vi "test-sync response for csm loop.vi"(8 "error in (no error)":errorcluster, 11 "TestCase in":refnum<class "testcase-csm loop support.lvclass">) -> (0 "error out":errorcluster, 3 "TestCase out":refnum<class "testcase-csm loop support.lvclass">)   [LabVIEW 2017, in "testcase-csm loop support.lvclass"]
uses:
  testcase-csm loop support.lvclass
  56d4bdba-c2f1-4b55-add1-7a078de9da03.vi
  ea54eaf7-6c78-4206-8259-080cdfbb85de.vi
  src/user.lib/_NEVSTOP/Communicable State Machine(CSM)/AdvanceAPI/CSM - Revert Arguments-Safe String.vi
  src/user.lib/_NEVSTOP/Communicable State Machine(CSM)/AdvanceAPI/CSM - Make String Arguments Safe.vi
  src/user.lib/_NEVSTOP/Communicable State Machine(CSM)/AdvanceAPI/CSM - Break Down Multiple States String.vi
  src/user.lib/_NEVSTOP/Communicable State Machine(CSM)/AdvanceAPI/CSM - Compact Multiple States.vi
  src/user.lib/_NEVSTOP/Communicable State Machine(CSM)/AdvanceAPI/CSM - Keywords.vi
  src/user.lib/_NEVSTOP/Communicable State Machine(CSM)/_Shared/Trim Single-line Text.vi
  <vilib>/addons/_JKI Toolkits/VI Tester/TestCase.llb/TestCase.lvclass
  src/user.lib/_NEVSTOP/Communicable State Machine(CSM)/Communicable State Machine.lvlib
  src/user.lib/_NEVSTOP/Communicable State Machine(CSM)/addons/Loop-Support/CSM Loop Support.lvlib
  C:/Program Files (x86)/National Instruments/LabVIEW 2017/vi.lib/addons/_JKI Toolkits/VI Tester/TestCase.llb/TestCase.lvclass
panel:
  out "State History":string
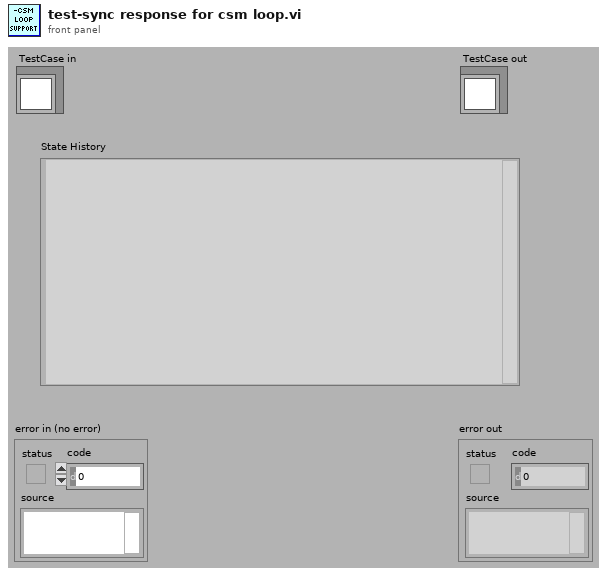
[diagram p1: front panel]
types:
  T1 = enum32{"Invalid", "Standard", "Closed", "Hidden", "Minimized", "Maximized"}
  T2 = enum32{"invalid app kind", "Development System", "Run Time System", "Student Edition", "Embedded LabVIEW", "Evaluation", "Custom"}
  T3 = typedef "Communicable State Machine.lvlib/_CSM_Response Source Message.ctl" = cluster{"‘State":string, "’Arguments":string, "’Error":errorcluster}
  T4 = cluster{"Current VI Reference":refnum<vi>, "Close Panel on Exit?":bool}
  T5 = cluster{"Core":cluster{"Current VI Reference":refnum<vi>, "Close Panel on Exit?":bool}, "diff":dbl, "time":timestamp}
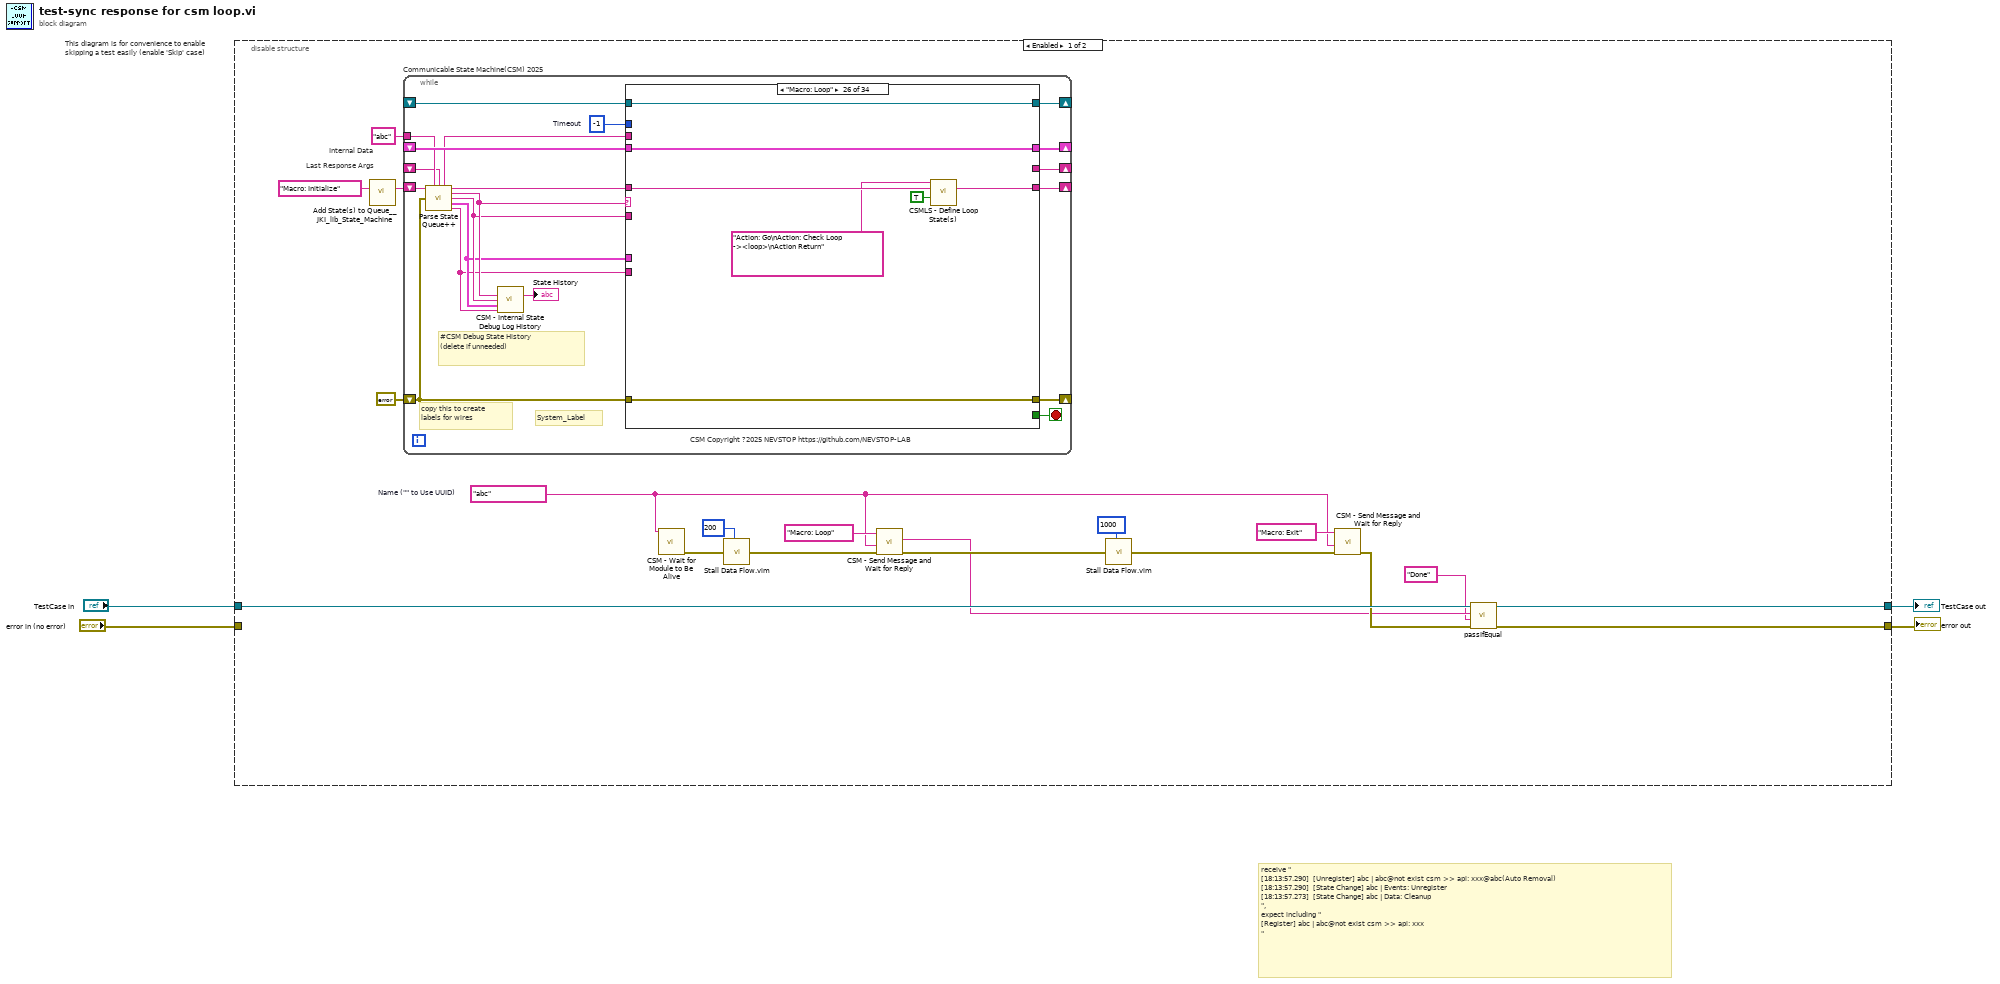
[diagram p0: block diagram]
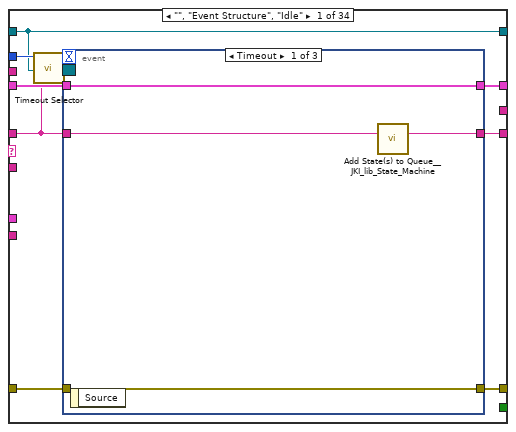
[diagram p2: hidden frame]
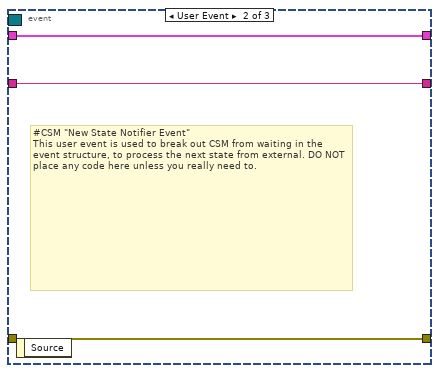
[diagram p3: hidden frame]
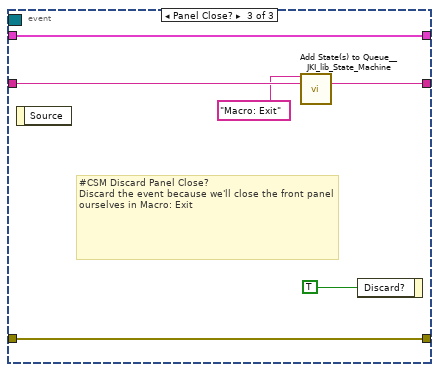
[diagram p4: hidden frame]
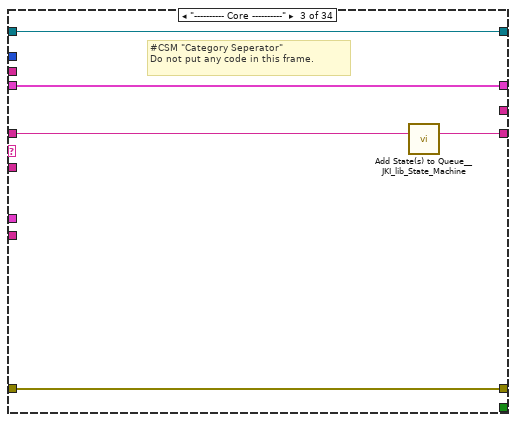
[diagram p6: hidden frame]
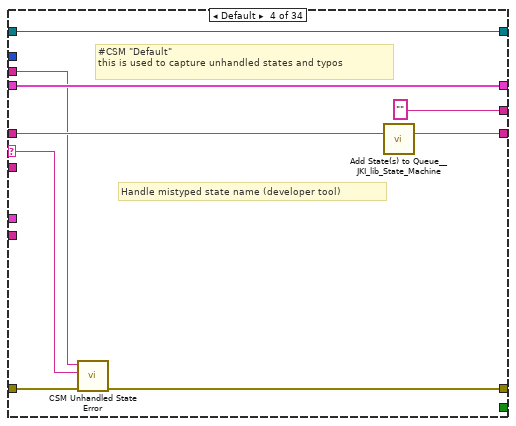
[diagram p7: hidden frame]
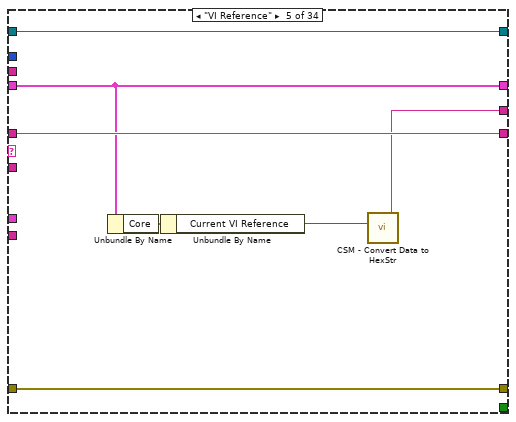
[diagram p8: hidden frame]
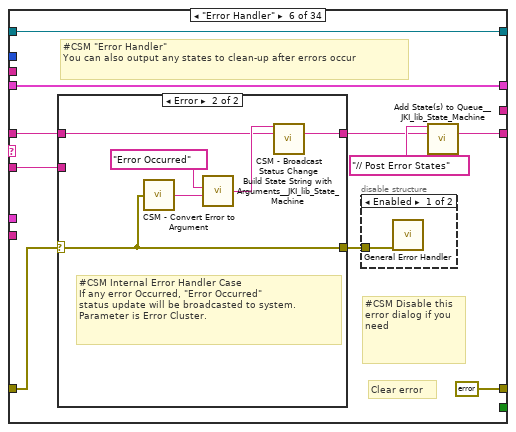
[diagram p9: hidden frame]
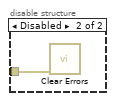
[diagram p10: hidden frame]
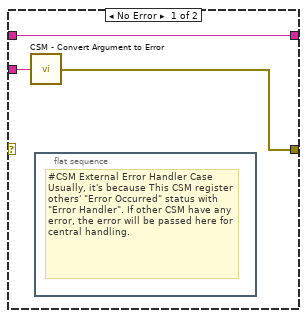
[diagram p11: hidden frame]
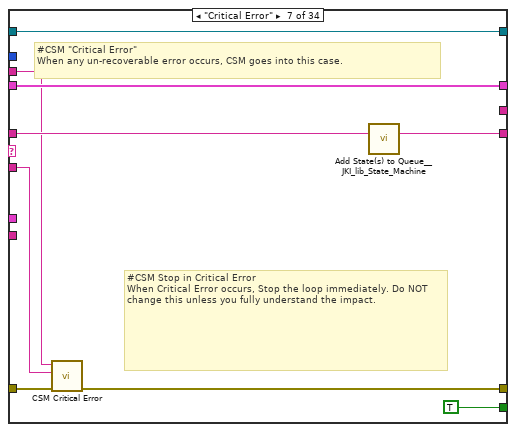
[diagram p12: hidden frame]
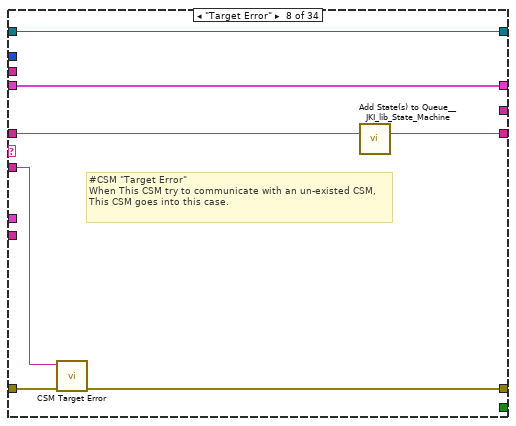
[diagram p13: hidden frame]
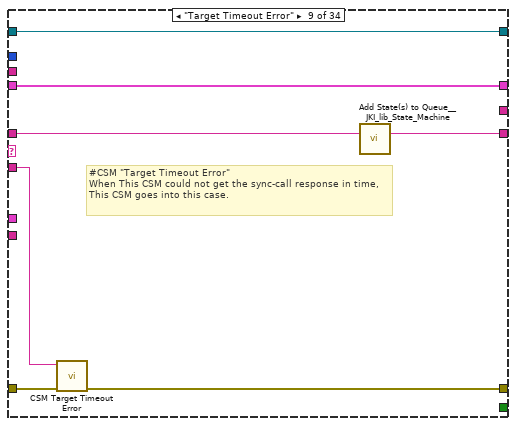
[diagram p14: hidden frame]
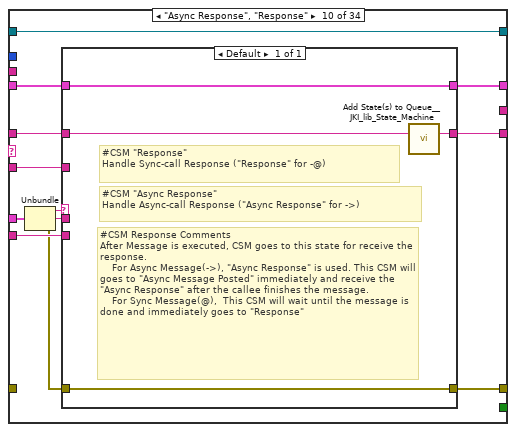
[diagram p15: hidden frame]
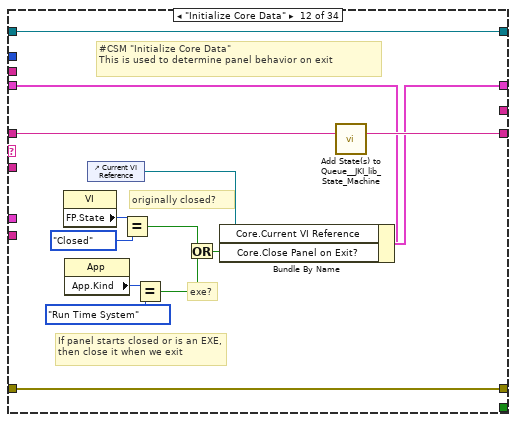
[diagram p17: hidden frame]
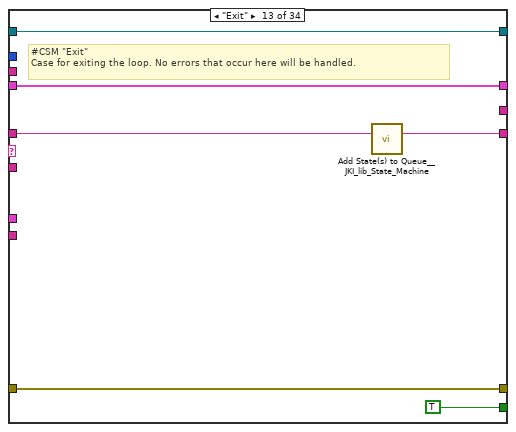
[diagram p18: hidden frame]
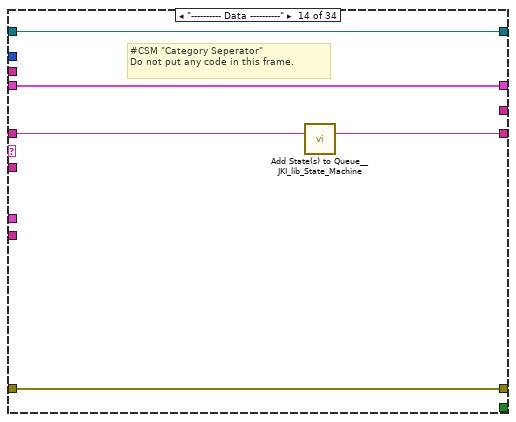
[diagram p19: hidden frame]
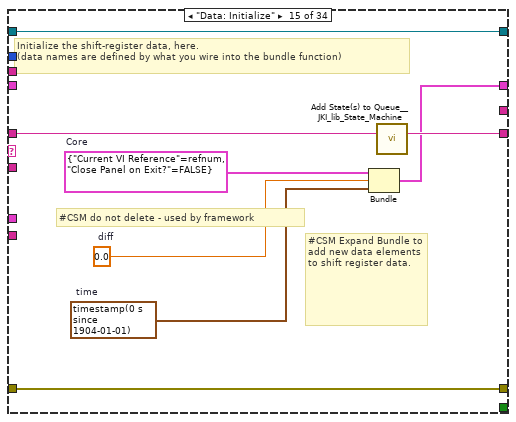
[diagram p20: hidden frame]
diagram:
  # "receive \"\n[18:13:57.290]  [Unregister] abc | abc@not exist csm >> api: xxx@abc(Auto Removal)\n[18:13:57.290]  [State Change] abc | Events: Unregister\n[18:13:57.273]  [State Change] abc | Data: Cleanup\n\", \nexpect including \"\n[Register] abc | abc@not exist csm >> api: xxx\n\""
  n1 = disable-structure "This diagram is for convenience to enable skipping a test easily (enable 'Skip' case)" shown="Enabled" {
    disable-tunnel: "TestCase in" -> [w14 w395]
    disable-tunnel: [w12 w393] -> w1
    disable-tunnel: [w11 w394] -> w3
    disable-tunnel: "error in (no error)" -> [_ w392]
    frame Enabled {
      w17 = "abc"  # Name ("" to Use UUID)
      # "Last Response Args"
      # "Internal Data"
      n2 = call <vilib>:"Add State(s) to Queue__JKI_lib_State_Machine.vi"("State(s) in (\"\")"="Macro: Initialize" ("Init State(\"Macro: Initialize\")")) -> ("States Out"=w21:string)  [unwired: 14 in]
      n3 = while "Communicable State Machine(CSM) 2025" {
        shift-right: [w38] -> _
        shift-left: _ -> [w37]
        shift-right: [w41] -> _
        shift-left: errorcluster {"status"=FALSE, "code"=0, "source"=""} ("error out") -> [w35]
        shift-right: [w40] -> _
        shift-left: w21 -> [w42]
        tunnel: "abc" ("Name (\"\" to Use UUID)") -> [w31]
        shift-right: [w34] -> _
        shift-left: _ -> [w25]
        shift-right: [w33] -> _
        shift-left: _ -> [w32]
        stop <- w39 stop-if-true
        w36 = -1  # Timeout
        # "#CSM Debug State History\n(delete if unneeded)"
        # "copy this to create labels for wires"
        # "System_Label"
        # "CSM Copyright ?2025 NEVSTOP https://github.com/NEVSTOP-LAB"
        n4 = call "Parse State Queue++.vi"("State Queue"=w42, "Name (\"\" to Use UUID)"=w31, "Response Arguments"=w25, "Previous Error"=w35) -> ("Name Used"=w26:string, "Remaining States"=w43:string, "Current State"=w30:string, "Arguments"=w29:string, "Additional Information"=w28:T3, "Source CSM"=w27:string)  [unwired: 6 in]
        n5 = call "CSM - Internal State Debug Log History.vi"("State"=w30, "Arguments (\"\")"=w29, ">> Response Source Message >>"=w28, "Source (\"\")"=w27) -> ("Debug Log"=→"State History":string)  [unwired: 11 in]
        n6 = case shown="\"Macro: Loop\"" w30 {
          selector: w30 -> [_ _ _ w77 _ _ _ _ _ _ _ _ _ _ _ _ _ _ _ _ _ _ _ _ _ _ _ _ _ _ _ _ w377 _]
          tunnel: w43 -> [w44 w68 w74 w82 w89 w95 w118 w124 w131 w140 w153 w168 w174 w179 w187 w194 w199 w206 w210 w216 w221 w228 w244 w314 w320 w327 w339 w342 w347 w353 w361 w368 w378 w390]
          tunnel: w29 -> [_ _ _ _ _ w94 w113 w123 w130 w139 _ _ _ _ _ _ _ _ _ _ _ w223 w238 _ _ _ _ _ _ w350 _ _ _ _]
          tunnel: w37 -> [w51 w67 w71 w80 w88 w99 w119 w126 w133 w142 w152 w161 w172 w176 _ w189 w196 w205 w209 w213 w219 w226 w240 w311 w317 w324 w336 w341 w346 w352 w358 w365 w374 w388]
          tunnel: [w50 w69 w72 w75 w90 errorcluster {"status"=FALSE, "code"=0, "source"=""} ("error out") w114 w121 w128 w145 w154 w165 w171 w177 w184 w190 w197 w200 w208 w214 w218 w224 w241 w312 w318 w325 w337 w343 w348 w354 w359 w366 w380 w391] -> w41
          tunnel: w35 -> [w49 w69 w72 w83 w90 w96 w120 w122 w129 _ w154 w165 w171 w177 w184 w191 w197 _ w211 w214 w218 w225 w242 w312 w318 w325 w337 w343 w348 w354 w359 w366 w380 w391]
          tunnel: [w52 w68 w73 w81 w89 w91 w117 w127 w134 w141 w153 w167 w173 w178 w186 w193 w198 w206 w210 w215 w220 w227 w243 w313 w319 w326 w338 w342 w347 w353 w360 w367 w381 w390] -> w40
          tunnel: [_ _ _ _ _ _ TRUE _ _ _ _ _ TRUE _ _ _ _ _ _ _ _ _ _ _ _ _ _ _ _ _ _ _ _ _] -> w39
          tunnel: [w48 w67 w71 w80 w88 w99 w119 w126 w133 w143 w152 w166 w172 w176 w185 w189 w196 w205 w209 w213 w219 w226 w240 w311 w317 w324 w336 w341 w346 w352 w358 w363 w370 w388] -> w38
          tunnel: w36 -> [w47 _ _ _ _ _ _ _ _ _ _ _ _ _ _ _ _ _ _ _ _ _ _ _ _ _ _ _ _ _ _ _ _ _]
          tunnel: w27 -> [_ _ _ _ _ _ _ _ _ w137 _ _ _ _ _ _ _ _ _ _ _ _ _ _ _ _ _ _ _ _ _ _ _ _]
          tunnel: w28 -> [_ _ _ _ _ _ _ _ _ w144 _ _ _ _ _ _ _ _ _ _ _ _ _ _ _ _ _ _ _ _ _ _ _ _]
          tunnel: [_ _ _ "" w84 _ _ _ _ _ _ _ _ _ _ _ _ _ _ _ _ _ _ _ _ _ _ _ "API1 Response" w349 _ _ _ "Done" ("HEX String (0-9,A-F)")] -> w34
          tunnel: [w46 w66 w70 w78 w87 w98 w115 w125 w132 w146 w151 w155 w169 w175 w180 w188 w195 w204 w207 w212 w217 w222 w237 w310 w315 w322 w329 w340 w345 w351 w357 w364 w379 w389] -> w33
          tunnel: w32 -> [w46 w66 w70 w78 w87 w98 w115 w125 w132 w146 w151 w155 w169 w175 w180 w188 w195 _ w207 w212 w217 w222 w237 w310 w315 w322 w329 w340 w345 w351 w357 w364 w379 w389]
          tunnel: w26 -> [_ _ _ w76 _ _ w112 _ _ _ _ _ _ _ _ _ _ w203 _ _ _ _ _ _ _ _ _ _ _ _ _ _ _ _]
          frame "", "Event Structure", "Idle" {
            n7 = call "Timeout Selector.vi"("Remaining States"=w44, "Timeout Expected"=w47) -> ("Timeout"=w45:i32)  [unwired: 5 in]
            n8 = event shown="[0] Timeout" {
              selector: w46 -> [_ _ _]
              dyn-events: _ -> [_ _ _]
              timeout: w45 -> [_ _ _]
              tunnel: w44 -> [w56 w58 w65]
              tunnel: [w55 w58 w64] -> w52
              tunnel: w51 -> [w53 w59 w62]
              tunnel: [w54 w57 w63] -> w50
              tunnel: w49 -> [w54 w57 w63]
              tunnel: [w53 w59 w62] -> w48
              event Timeout {
                n9 = event-data() -> ()  [unwired: 1 in, 1 out]
                n10 = call <vilib>:"Add State(s) to Queue__JKI_lib_State_Machine.vi"("State(s) in (\"\")"=w56) -> ("States Out"=w55:string)  [unwired: 14 in]
              }
              event User Event {
                # "#CSM \"New State Notifier Event\"\nThis user event is used to break out CSM from waiting in the event structure, to process the next state from external. DO NOT place any code here unless you really need to."
                n11 = event-data() -> ()  [unwired: 1 in, 1 out]
              }
              event Panel Close? {
                # "#CSM Discard Panel Close?\nDiscard the event because we'll close the front panel ourselves in Macro: Exit"
                n12 = event-data() -> ()  [unwired: 1 in, 1 out]
                n13 = call <vilib>:"Add State(s) to Queue__JKI_lib_State_Machine.vi"("State(s) in Front (\"\")"="Macro: Exit", "State(s) in (\"\")"=w65) -> ("States Out"=w64:string)  [unwired: 13 in]
                n14 = event-data("Discard?"=TRUE) -> ()  [unwired: 1 in, 1 out]
              }
            }
          }
          frame "CSM Documentation" {
            # "#CSM README FIRST\n\nCommunicable State Machine(CSM) is a LabVIEW application framework that builds upon JKI State Machine(JKISM). It follows the pattern of JKISM and extends the keywords to describe message communication between modules, including concepts such as Sync-Message, Async-Message, Subscription/Unsubscription of status - essential elements for creating reusable code modules. For more information, please visit the CSM wiki: https://nevstop-lab.github.io/CSM-Wiki/\n\nFor instructions on JKI State Machine, visit: http://jki.net/state-machine/\nFor information about CSM, visit: https://github.com/NEVSTOP-LAB"
            # "#CSM \"Documentation\"\nCase for holding CSM Documenation"
          }
          frame "---------- Core ----------" {
            # "#CSM \"Category Seperator\"\nDo not put any code in this frame."
            n15 = call <vilib>:"Add State(s) to Queue__JKI_lib_State_Machine.vi"("State(s) in (\"\")"=w74) -> ("States Out"=w73:string)  [unwired: 14 in]
          }
          frame Default {
            # "#CSM \"Default\"\nthis is used to capture unhandled states and typos"
            # "Handle mistyped state name (developer tool)"
            n16 = call "CSM Unhandled State Error.vi"("error in (no error)"=w83, "Undefined State"=w77, "CSM Name"=w76) -> ("error out"=w75:errorcluster)  [unwired: 8 in]
            n17 = call <vilib>:"Add State(s) to Queue__JKI_lib_State_Machine.vi"("State(s) in (\"\")"=w82) -> ("States Out"=w81:string)  [unwired: 14 in]
          }
          frame "VI Reference" {
            n18 = Unbundle By Name(w88) -> ("Core"=w86:T4)
            n19 = Unbundle By Name(w86) -> ("Current VI Reference"=w85:refnum<vi>)
            n20 = call "CSM - Convert Data to HexStr.vi"("Variant"=w85) -> ("HEX String (0-9,A-F)"=w84:string)  [unwired: 8 in]
          }
          frame "Error Handler" {
            # "#CSM Disable this error dialog if you need"
            # "#CSM \"Error Handler\"\nYou can also output any states to clean-up after errors occur"
            # "Clear error"
            n21 = case shown="Error" w96 {
              selector: w96 -> [_ w106]
              tunnel: [w105 w108] -> w92
              tunnel: w95 -> [w105 w107]
              tunnel: w94 -> [w104 _]
              tunnel: [w103 w106] -> w97
              frame No Error {
                n22 = call "CSM - Convert Argument to Error.vi"("Argument"=w104) -> ("Error"=w103:errorcluster)  [unwired: 4 in]
                n23 = flat-sequence {
                  frame #0 {
                    # "#CSM External Error Handler Case\nUsually, it's because This CSM register others' \"Error Occurred\" status with \"Error Handler\". If other CSM have any error, the error will be passed here for central handling."
                  }
                }
              }
              frame Error {
                # "#CSM Internal Error Handler Case \nIf any error Occurred, \"Error Occurred\" \nstatus update will be broadcasted to system.\nParameter is Error Cluster."
                n24 = call "CSM - Convert Error to Argument.vi"("Error"=w106) -> ("Argument"=w110:string)  [unwired: 4 in]
                n25 = call <vilib>:"Build State String with Arguments__JKI_lib_State_Machine.vi"("Arguments (\"\")"=w110, "State"="Error Occurred" ("Status with Arguments")) -> ("State with Arguments"=w109:string)  [unwired: 4 in]
                n26 = call "CSM - Broadcast Status Change.vi"("Status With Arguments"=w109, "State Queue"=w107) -> ("Remaining States"=w108:string)  [unwired: 13 in]
              }
            }
            n27 = disable-structure shown="Enabled" {
              disable-tunnel: w97 -> [w101 w102]
              frame Enabled {
                n28 = call <vilib>:"General Error Handler.vi"("error in (no error)"=w101) -> ()  [unwired: 10 in, 5 out]
              }
              frame Disabled {
                n29 = call <vilib>:"Clear Errors.vi"("error in (no error)"=w102) -> ()  [unwired: 5 in, 2 out]
              }
            }
            n30 = call <vilib>:"Add State(s) to Queue__JKI_lib_State_Machine.vi"("State(s) in Front (\"\")"="// Post Error States", "State(s) in (\"\")"=w92) -> ("States Out"=w91:string)  [unwired: 13 in]
          }
          frame "Critical Error" {
            # "#CSM Stop in Critical Error\nWhen Critical Error occurs, Stop the loop immediately. Do NOT change this unless you fully understand the impact."
            # "#CSM \"Critical Error\"\nWhen any un-recoverable error occurs, CSM goes into this case."
            n31 = call "CSM Critical Error.vi"("error in (no error)"=w120, "Arugments (As Reason)"=w113, "CSM Name"=w112) -> ("error out"=w114:errorcluster)  [unwired: 8 in]
            n32 = call <vilib>:"Add State(s) to Queue__JKI_lib_State_Machine.vi"("State(s) in (\"\")"=w118) -> ("States Out"=w117:string)  [unwired: 14 in]
          }
          frame "Target Error" {
            # "#CSM \"Target Error\"\nWhen This CSM try to communicate with an un-existed CSM, This CSM goes into this case."
            n33 = call "CSM Target Error.vi"("error in (no error)"=w122, "Arguments (As CSM Name)"=w123) -> ("error out"=w121:errorcluster)  [unwired: 9 in]
            n34 = call <vilib>:"Add State(s) to Queue__JKI_lib_State_Machine.vi"("State(s) in (\"\")"=w124) -> ("States Out"=w127:string)  [unwired: 14 in]
          }
          frame "Target Timeout Error" {
            # "#CSM \"Target Timeout Error\"\nWhen This CSM could not get the sync-call response in time, This CSM goes into this case."
            n35 = call "CSM Target Timeout Error.vi"("error in (no error)"=w129, "Arguments (As CSM Name)"=w130) -> ("error out"=w128:errorcluster)  [unwired: 9 in]
            n36 = call <vilib>:"Add State(s) to Queue__JKI_lib_State_Machine.vi"("State(s) in (\"\")"=w131) -> ("States Out"=w134:string)  [unwired: 14 in]
          }
          frame "Async Response", "Response" {
            n37 = Unbundle(w144) -> ("‘State"=w138:string, "’Arguments"=w136:string, "’Error"=w135:errorcluster)
            n38 = case shown="Default" w138 {
              tunnel: [w150] -> w145
              tunnel: w135 -> [w150]
              tunnel: [w149] -> w143
              tunnel: w142 -> [w149]
              tunnel: [w147] -> w141
              tunnel: w140 -> [w148]
              tunnel: w139 -> [_]
              tunnel: w137 -> [_]
              tunnel: w136 -> [_]
              frame Default {
                # "#CSM Response Comments\nAfter Message is executed, CSM goes to this state for receive the response.\n    For Async Message(->), \"Async Response\" is used. This CSM will goes to \"Async Message Posted\" immediately and receive the \"Async Response\" after the callee finishes the message.\n    For Sync Message(@),  This CSM will wait until the message is done and immediately goes to \"Response\""
                # "#CSM \"Async Response\"\nHandle Async-call Response (\"Async Response\" for ->)"
                # "#CSM \"Response\"\nHandle Sync-call Response (\"Response\" for -@)"
                n39 = call <vilib>:"Add State(s) to Queue__JKI_lib_State_Machine.vi"("State(s) in (\"\")"=w148) -> ("States Out"=w147:string)  [unwired: 14 in]
              }
            }
          }
          frame "Async Message Posted" {
            # "#CSM \"Async Message Posted\"\nAfter Async Message is posted (-> or ->| ), CSM goes to this state for post-action.\nYou can use Argument - State to tell which Async Message is called."
          }
          frame "Initialize Core Data" {
            # "#CSM \"Initialize Core Data\"\nThis is used to determine panel behavior on exit"
            # "originally closed?"
            # "exe?"
            # "If panel starts closed or is an EXE, then close it when we exit"
            n40 = property class="VI"() -> ("FP.State"=w158:T1)  [unwired: 2 in, 2 out]
            n41 = property class="App"() -> ("App.Kind"=w164:T2)  [unwired: 2 in, 2 out]
            n42 = control-ref of="Current VI Reference"() -> (w159:refnum<vi>)
            n43 = Equal?(x=w158, y=T1."Closed" ("Front Panel Window:State")) -> (x = y?=w156:bool)
            n44 = Equal?(x=w164, y=T2."Run Time System" ("Application:Kind")) -> (x = y?=w162:bool)
            n45 = Or(x=w156, y=w162) -> (x .or. y?=w160:bool)
            n46 = Bundle By Name(cluster=w161, "Core.Current VI Reference"=w159, "Core.Close Panel on Exit?"=w160) -> (w166:T5)
            n47 = call <vilib>:"Add State(s) to Queue__JKI_lib_State_Machine.vi"("State(s) in (\"\")"=w168) -> ("States Out"=w167:string)  [unwired: 14 in]
          }
          frame "Exit" {
            # "#CSM \"Exit\"\nCase for exiting the loop. No errors that occur here will be handled."
            n48 = call <vilib>:"Add State(s) to Queue__JKI_lib_State_Machine.vi"("State(s) in (\"\")"=w174) -> ("States Out"=w173:string)  [unwired: 14 in]
          }
          frame "---------- Data ----------" {
            # "#CSM \"Category Seperator\"\nDo not put any code in this frame."
            n49 = call <vilib>:"Add State(s) to Queue__JKI_lib_State_Machine.vi"("State(s) in (\"\")"=w179) -> ("States Out"=w178:string)  [unwired: 14 in]
          }
          frame "Data: Initialize" {
            w181 = T4 {"Current VI Reference"=refnum, "Close Panel on Exit?"=FALSE}  # Core
            w183 = 0.0  # diff
            w182 = timestamp(0 s since 1904-01-01)  # time
            # "#CSM do not delete - used by framework"
            # "#CSM Expand Bundle to add new data elements to shift register data."
            # "Initialize the shift-register data, here.\n(data names are defined by what you wire into the bundle function)"
            n50 = Bundle("Core"=w181, "diff"=w183, "time"=w182) -> (w185:T5)  [unwired: 1 in]
            n51 = call <vilib>:"Add State(s) to Queue__JKI_lib_State_Machine.vi"("State(s) in (\"\")"=w187) -> ("States Out"=w186:string)  [unwired: 14 in]
          }
          frame "Data: Cleanup" {
            # "Cleanup any data and references, here.\n(this is called automatically, by the Macro: Exit)"
            n52 = Unbundle By Name(w189) -> ("Core.Current VI Reference"=w192:refnum<vi>)
            n53 = Close Reference(reference=w192, error in (no error)=w191) -> (error out=w190:errorcluster)
            n54 = call <vilib>:"Add State(s) to Queue__JKI_lib_State_Machine.vi"("State(s) in (\"\")"=w194) -> ("States Out"=w193:string)  [unwired: 14 in]
          }
          frame "---------- Events ----------" {
            # "#CSM \"Category Seperator\"\nDo not put any code in this frame."
            n55 = call <vilib>:"Add State(s) to Queue__JKI_lib_State_Machine.vi"("State(s) in (\"\")"=w199) -> ("States Out"=w198:string)  [unwired: 14 in]
          }
          frame "Events: Register" {
            # "#CSM \"Events: Register\"\nRegister user event. New Message Event is registered to break CSM waiting in event structure by default."
            # "#CSM Register New Message Event\nRegister message event to break Waiting in Event structure."
            n56 = call "CSM - Get New State Notifier Event.vi"("Name (\"\" to Use UUID)"=w203) -> ("error out"=w201:errorcluster, "New State Notifier Event"=w202:refnum<user-event>)  [unwired: 9 in]
            n57 = register-events(error in=w201, w202) -> (reference out=w204:refnum<event-registration>, error out=w200:errorcluster)  [unwired: 1 in]
          }
          frame "Events: Unregister" {
            # "#CSM \"Events: Unregister\"\nUnregister user event."
            n58 = Unregister For Events(event registration refnum=w207, error in=w211) -> (error out=w208:errorcluster)
          }
          frame "---------- UI ----------" {
            # "#CSM \"Category Seperator\"\nDo not put any code in this frame."
            n59 = call <vilib>:"Add State(s) to Queue__JKI_lib_State_Machine.vi"("State(s) in (\"\")"=w216) -> ("States Out"=w215:string)  [unwired: 14 in]
          }
          frame "UI: Initialize" {
            # "#CSM \"UI: Initialize\"\nInitialize the User Interface, here.\n(this is called automatically, by the Macro: Init)"
            n60 = call <vilib>:"Add State(s) to Queue__JKI_lib_State_Machine.vi"("State(s) in (\"\")"=w221) -> ("States Out"=w220:string)  [unwired: 14 in]
          }
          frame "UI: Cursor Set" {
            # "#CSM \"UI: Cursor Set\"\nSet and Unset Cursor Busy.\n(Usage: \"UI: Cursor Set >> Busy|Idle\")"
            # "Argument"
            n61 = disable-structure shown="Default" {
              disable-tunnel: w225 -> [w231 w236]
              disable-tunnel: [w230 w236] -> w224
              disable-tunnel: w223 -> [w229 _]
              frame condition #0 (active) {
                n62 = case shown="\"Idle\", Default" w229 {
                  tunnel: w231 -> [w233 w235]
                  tunnel: [w232 w234] -> w230
                  frame "Idle", Default {
                    n63 = call <vilib>:"Unset Busy.vi"("error in (no error)"=w233) -> ("error out"=w232:errorcluster)  [unwired: 10 in]
                  }
                  frame "Busy" {
                    n64 = call <vilib>:"Set Busy.vi"("error in (no error)"=w235) -> ("error out"=w234:errorcluster)  [unwired: 9 in, 1 out]
                  }
                }
              }
              frame condition #1 {
              }
            }
            n65 = call <vilib>:"Add State(s) to Queue__JKI_lib_State_Machine.vi"("State(s) in (\"\")"=w228) -> ("States Out"=w227:string)  [unwired: 14 in]
          }
          frame "UI: Front Panel State" {
            # "#CSM \"UI: Front Panel State\"\nSet Front Panel Open or Closed\n(Usage: \"UI: Front Panel State >> Open|Close\")"
            # "Argument"
            n66 = Unbundle By Name(w240) -> ("Core.Current VI Reference"=w239:refnum<vi>)
            n67 = call <vilib>:"Add State(s) to Queue__JKI_lib_State_Machine.vi"("State(s) in (\"\")"=w244) -> ("States Out"=w243:string)  [unwired: 14 in]
            n68 = case shown="\"Close\", \"Closed\"" w238 {
              tunnel: w242 -> [w250 w265 w276 w289 w302]
              tunnel: [w252 w266 w278 w291 w304] -> w241
              tunnel: w239 -> [w251 w263 w277 w290 w303]
              frame "Open", "Standard", Default {
                w245 = T1."Standard" ("State")
                n69 = property class="VI"(reference=w251, error in=w250) -> (reference out=w248:refnum<vi>, error out=w249:errorcluster, "FP.State"=w247:T1)
                n70 = Not Equal?(x=w247, y=w245) -> (x != y?=w246:bool)
                n71 = case shown="True" w246 {
                  tunnel: [w256 w258] -> w252
                  tunnel: w249 -> [w255 w258]
                  tunnel: w248 -> [w254 _]
                  tunnel: w245 -> [w253 _]
                  frame True {
                    n72 = invoke class="VI" method="FP.Open"(reference=w254, error in=w255, "Activate"=TRUE, "State"=w253) -> (error out=w256:errorcluster)  [unwired: 1 in, 4 out]
                  }
                  frame False {
                  }
                }
              }
              frame "Close", "Closed" {
                n73 = property class="VI"(reference=w263, error in=w265) -> (reference out=w262:refnum<vi>, error out=w264:errorcluster, "FP.State"=w260:T1)
                n74 = Not Equal?(x=w260, y=T1."Closed" ("Front Panel Window:State")) -> (x != y?=w259:bool)
                n75 = case shown="False" w259 {
                  tunnel: [w267 w270] -> w266
                  tunnel: w264 -> [w267 w269]
                  tunnel: w262 -> [_ w268]
                  frame False {
                  }
                  frame True {
                    n76 = invoke class="VI" method="FP.Close"(reference=w268, error in=w269) -> (error out=w270:errorcluster)  [unwired: 1 in, 2 out]
                  }
                }
              }
              frame "Hidden", "Hide" {
                w271 = T1."Hidden" ("State")
                n77 = property class="VI"(reference=w277, error in=w276) -> (reference out=w274:refnum<vi>, error out=w275:errorcluster, "FP.State"=w273:T1)
                n78 = Not Equal?(x=w273, y=w271) -> (x != y?=w272:bool)
                n79 = case shown="True" w272 {
                  tunnel: [w282 w283] -> w278
                  tunnel: w275 -> [w281 w283]
                  tunnel: w274 -> [w280 _]
                  tunnel: w271 -> [w279 _]
                  frame True {
                    n80 = invoke class="VI" method="FP.Open"(reference=w280, error in=w281, "State"=w279) -> (error out=w282:errorcluster)  [unwired: 2 in, 4 out]
                  }
                  frame False {
                  }
                }
              }
              frame "Minimize", "Minimized" {
                w284 = T1."Minimized" ("State")
                n81 = property class="VI"(reference=w290, error in=w289) -> (reference out=w287:refnum<vi>, error out=w288:errorcluster, "FP.State"=w286:T1)
                n82 = Not Equal?(x=w286, y=w284) -> (x != y?=w285:bool)
                n83 = case shown="True" w285 {
                  tunnel: [w295 w296] -> w291
                  tunnel: w288 -> [w294 w296]
                  tunnel: w287 -> [w293 _]
                  tunnel: w284 -> [w292 _]
                  frame True {
                    n84 = invoke class="VI" method="FP.Open"(reference=w293, error in=w294, "State"=w292) -> (error out=w295:errorcluster)  [unwired: 2 in, 4 out]
                  }
                  frame False {
                  }
                }
              }
              frame "Maximize", "Maximized" {
                w297 = T1."Maximized" ("State")
                n85 = property class="VI"(reference=w303, error in=w302) -> (reference out=w300:refnum<vi>, error out=w301:errorcluster, "FP.State"=w299:T1)
                n86 = Not Equal?(x=w299, y=w297) -> (x != y?=w298:bool)
                n87 = case shown="True" w298 {
                  tunnel: [w308 w309] -> w304
                  tunnel: w301 -> [w307 w309]
                  tunnel: w300 -> [w306 _]
                  tunnel: w297 -> [w305 _]
                  frame True {
                    n88 = invoke class="VI" method="FP.Open"(reference=w306, error in=w307, "State"=w305) -> (error out=w308:errorcluster)  [unwired: 2 in, 4 out]
                  }
                  frame False {
                  }
                }
              }
            }
          }
          frame "---------- Macro ----------" {
            # "#CSM \"Category Seperator\"\nDo not put any code in this frame."
            n89 = call <vilib>:"Add State(s) to Queue__JKI_lib_State_Machine.vi"("State(s) in (\"\")"=w314) -> ("States Out"=w313:string)  [unwired: 14 in]
          }
          frame "Macro: Initialize" {
            w316 = "Data: Initialize\nInitialize Core Data\nEvents: Register\nUI: Initialize\nUI: Front Panel State >> Open"  # Data: Initialize Initialize Core Data Events: Register UI: Initialize UI: Front Panel State >> Open
            # "#CSM \"Macro: Initialize\"\nInitialization Macro (This is called once, when the VI starts)"
            n90 = call <vilib>:"Add State(s) to Queue__JKI_lib_State_Machine.vi"("State(s) in Front (\"\")"=w316, "State(s) in (\"\")"=w320) -> ("States Out"=w319:string)  [unwired: 13 in]
          }
          frame "Macro: Loop" {
            n91 = call "CSMLS - Define Loop State(s).vi"("Loop States"="Action: Go\nAction: Check Loop -><loop>\nAction Return", "States Queue"=w327, "Add to Front? (F)"=TRUE ("Front(T)/Back(F)")) -> ("Remaining States"=w326:string)  [unwired: 12 in]
          }
          frame "Macro: Exit" {
            # "#CSM \"Macro: Exit\"\nExit Macro (This is called once, when the VI exits)"
            n92 = Unbundle By Name(w336) -> ("Core.Close Panel on Exit?"=w335:bool)
            n93 = Select(t="UI: Front Panel State >> Close", s=w335, f="") -> (s? t:f=w332:string)
            n94 = call <vilib>:"Add State(s) to Queue__JKI_lib_State_Machine.vi"("State(s) in Front (\"\")"="//Exit Sub-Modules ", "State(s) in (\"\")"=w332, "State(s) at Back (\"\")"="Data: Cleanup\nEvents: Unregister\nExit") -> ("States Out"=w330:string)  [unwired: 12 in]
            n95 = call <vilib>:"Add State(s) to Queue__JKI_lib_State_Machine.vi"("State(s) in Front (\"\")"=w330, "State(s) in (\"\")"=w339) -> ("States Out"=w338:string)  [unwired: 13 in]
          }
          frame "---------- API ----------" {
            # "#CSM \"Category Seperator\"\nDo not put any code in this frame."
          }
          frame "API: API1" {
            # "#CSM API Example\nCopy/Rename this case for your own API"
            # "#CSM Response\nConnect this to return the response of your API"
            # "#CSM >> Source CSM >>\nIf you need to tell who triggered this state , use this string. If it's this case itself, this string is \"\"."
            # "#CSM >> Arguments >>\nDeal with the parameter if any"
          }
          frame "API: API2" {
            # "#CSM API Example\nCopy/Rename this case for your own API"
            # "unpack Hex String  to Variant\nif complex parameter is needed."
            n96 = call "CSM - Convert HexStr to Data.vi"("HEX String"=w350) -> ()  [unwired: 7 in, 2 out]
            n97 = disable-structure shown="Disabled" {
              disable-tunnel: [w355 "API2 Response"] -> w349
              frame Disabled {
                # "pack variant to hexstr \nif complex response is needed."
                # "complex Response"
                n98 = call "CSM - Convert Data to HexStr.vi"() -> ("HEX String (0-9,A-F)"=w355:string)  [unwired: 9 in]
              }
              frame Enabled {
              }
            }
          }
          frame "---------- Action ----------" {
            # "#CSM \"Category Seperator\"\nDo not put any code in this frame."
            n99 = call <vilib>:"Add State(s) to Queue__JKI_lib_State_Machine.vi"("State(s) in (\"\")"=w361) -> ("States Out"=w360:string)  [unwired: 14 in]
          }
          frame "Action: Go" {
            n100 = Get Date/Time In Seconds() -> (seconds since 1Jan1904=w362:timestamp)
            n101 = Bundle By Name(cluster=w365, "time"=w362) -> (w363:T5)
            n102 = call <vilib>:"Add State(s) to Queue__JKI_lib_State_Machine.vi"("State(s) in (\"\")"=w368) -> ("States Out"=w367:string)  [unwired: 14 in]
          }
          frame "Action: Check Loop" {
            n103 = Unbundle By Name(w374) -> ("time"=w373:timestamp)
            n104 = Wait (ms)(milliseconds to wait=u32 100) -> ()  [unwired: 1 out]
            n105 = Get Date/Time In Seconds() -> (seconds since 1Jan1904=w375:timestamp)
            n106 = Subtract(x=w375, y=w373) -> (x-y=w369:dbl)
            n107 = Greater?(x=w369, y=3.0) -> (0:w371:bool)
            n108 = case shown="False" w371 {
              tunnel: [w385 w386] -> w381
              tunnel: w378 -> [w384 w386]
              tunnel: w377 -> [w383 _]
              frame False {
                n109 = call "CSMLS - Append Continuous State.vi"("Loop State(s) And Arguments"="" ("Loop State(s) and Arguments"), "Continous State"=w383, "States Queue"=w384) -> ("Remaining States"=w385:string)  [unwired: 8 in]
              }
              frame True {
              }
            }
            n110 = Bundle By Name(cluster=w374, "diff"=w369) -> (w370:T5)
          }
          frame "Action Return" {
          }
        }
      }
      n111 = call "CSM - Wait for Module to Be Alive.vi"("CSM Name"=w17) -> ("error out"=w16:errorcluster)  [unwired: 12 in, 2 out]
      n112 = call "Stall Data Flow.vim"("value in"=w16, "milliseconds to wait"=u32 200) -> ("value out"=w6:errorcluster)  [unwired: 1 out]
      n113 = call "CSM - Send Message and Wait for Reply.vi"("Error In (No Error)"=w6, "Target Module"=w17, "State"="Macro: Loop") -> ("error out"=w15:errorcluster, "Response"=w10:string)  [unwired: 6 in, 1 out]
      n114 = call "Stall Data Flow.vim"("value in"=w15, "milliseconds to wait"=u32 1000) -> ("value out"=w8:errorcluster)  [unwired: 1 out]
      n115 = call "CSM - Send Message and Wait for Reply.vi"("Error In (No Error)"=w8, "Target Module"=w17, "State"="Macro: Exit") -> ("error out"=w13:errorcluster)  [unwired: 6 in, 2 out]
      n116 = call-dynamic "passIfEqual.vi"("error in (no error)"=w13, "y"="Done" ("HEX String (0-9,A-F)"), "x"=w10, "TestCase in"=w14) -> ("error out"=w11:errorcluster, "TestCase out"=w12:refnum<class "testcase-csm loop support.lvclass">)  [unwired: 6 in]
    }
    frame Disabled {
      # "skip test result while test is under development"
      n117 = call <vilib>:"skip.vi"("error in (no error)"=w392, "TestCase in"=w395) -> ("error out"=w394:errorcluster, "TestCase out"=w393:refnum<class "testcase-csm loop support.lvclass">)  [unwired: 8 in]
    }
  }
  "error out" <- w3
  "TestCase out" <- w1
